vi "WeatherMapAPI_CurrentWeather-Main.vi"() -> (0 "error out":errorcluster, 1 "URL":string, 3 "WeatherMap Current Weather Data":T1)   [LabVIEW 2021]
doc: "Developed By: J Branch\nLast Update: 9/4/2022\n\nDescription: Returns the current weather data to the front panel using the WeatherMap API via HTTP request. The user will need to first navigate to https://openweathermap.org to create an account to get an API key to use the program.\n\nInputs: Zip Code, Country Code\n\nOutput: WeatherMap Current Weather Data Cluster\n\nTo Run: On the block diagram enter the user's API Key into the string text box labelled API Key. Enter the Zip Code and Country Code (us default) in the front panel and select GET Data to execute the API call, the API JSON response will be parsed in the background inside the sub-VIs and formatted to populate the WeatherMap Current Weather Data cluster. \n\nThe Zip Code and County Code can be modified during run-time. \n\nSelect QUIT to terminate the program."
uses:
  <vilib>/httpClient/LabVIEWHTTPClient.lvlib
panel:
  in  "Tab Control":enum32{"User Params", "Internal Params"}(tab)
  out "UserMsg":string
  in  "GetDataButton":bool
  in  "QuitProgramButton":bool
  in  "Zip Code":string
  in  "Country Code":string="us"
  out "HTTP Headers":string
  out "HTTP Body":string
  out "API Key":string="a672f85a4c2930ce00107a5976b7c754"
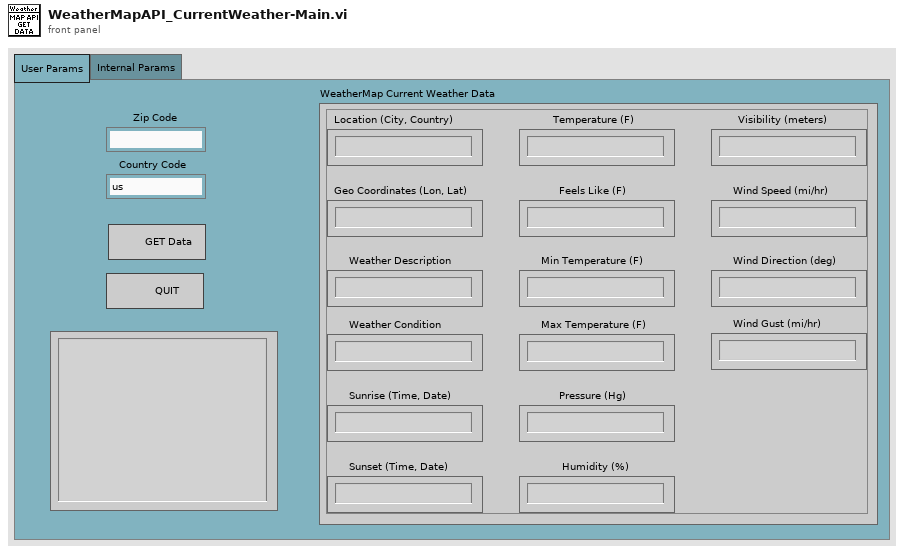
[diagram p1: front panel]
types:
  T1 = cluster{"Location (City, Country)":string, "Geo Coordinates (Lon, Lat)":string, "Weather Description ":string, "Weather Condition":string, "Temperature (F)":string, "Feels Like (F)":string, "Min Temperature (F)":string, "Max Temperature (F)":string, "Pressure (Hg) ":string, "Humidity (%)":string, "Visibility (meters)":string, "Wind Speed (mi/hr)":string, "Wind Direction (deg)":string, "Sunrise (Time, Date)":string, "Sunset (Time, Date)":string, "Wind Gust (mi/hr) ":string}
  T2 = enum8{"Enabled", "Disabled", "Disabled and Grayed Out"}
  T3 = typedef "LabVIEWHTTPClient.lvlib/ClientHandle.ctl" = refnum<k1>
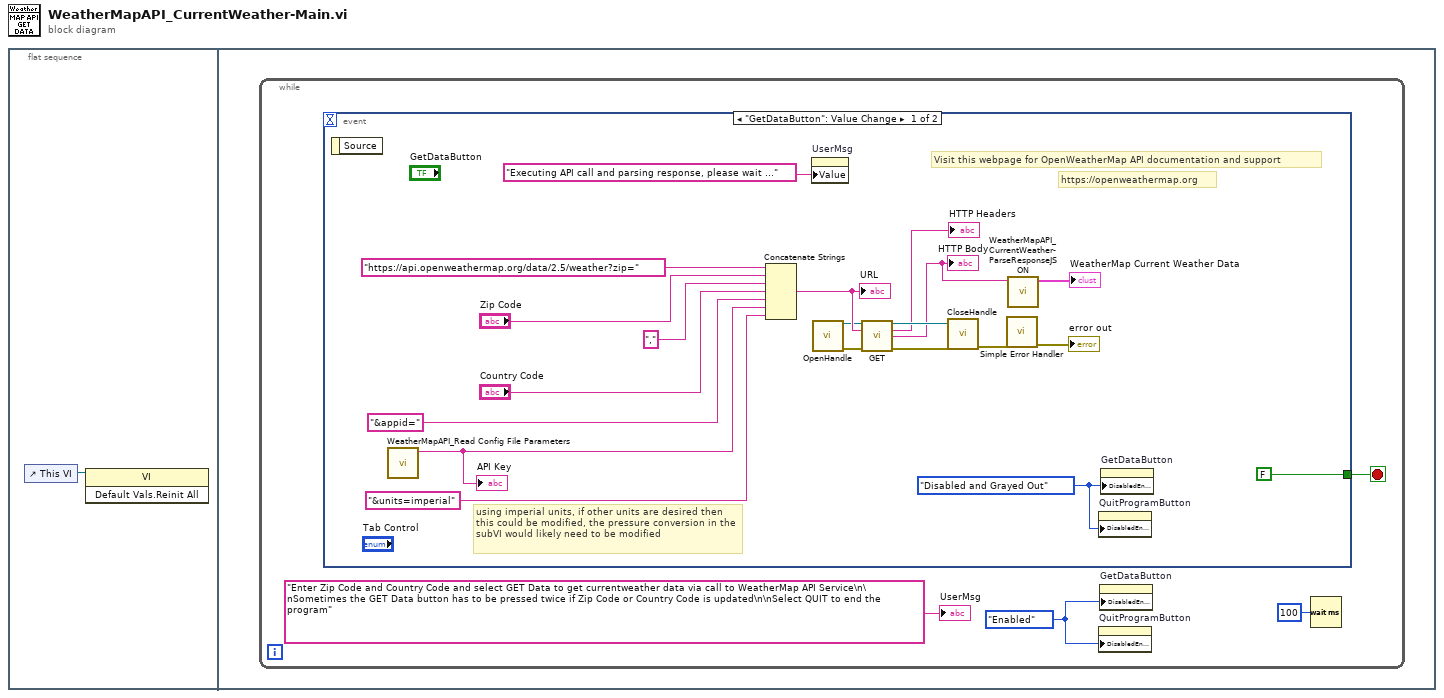
[diagram p0: block diagram]
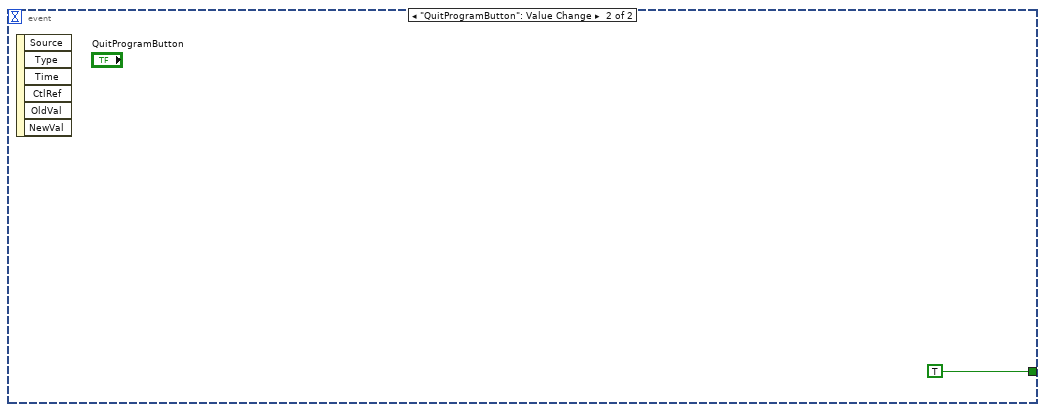
[diagram p2: hidden frame]
diagram:
  n1 = flat-sequence {
    frame #0 {
      n2 = control-ref of="This VI"() -> (w1:refnum<vi>)
      n3 = invoke class="VI" method="Default Vals.Reinit All"(reference=w1) -> ()  [unwired: 2 in, 3 out]
    }
    frame #1 {
      n4 = while {
        stop <- w3 stop-if-true
        w2 = T2."Enabled" ("Disabled")
        n5 = event shown="[0] \"GetDataButton\": Value Change" {
          selector: _ -> [_ _]
          dyn-events: _ -> [_ _]
          timeout: _ -> [_ _]
          tunnel: [FALSE TRUE] -> w3
          event "GetDataButton": Value Change {
            w15 = T2."Disabled and Grayed Out" ("Disabled")
            # "using imperial units, if other units are desired then this could be modified, the pressure conversion in the subVI would likely need to be modified"
            # "Visit this webpage for OpenWeatherMap API documentation and support"
            # "https://openweathermap.org"
            n6 = event-data() -> ()  [unwired: 1 in, 1 out]
            n7 = call "WeatherMapAPI_Read Config File Parameters.vi"() -> ("API Key out"=w6:string)  [unwired: 10 in, 1 out]
            "API Key" <- w6
            n8 = Concatenate Strings("https://api.openweathermap.org/data/2.5/weather?zip=", "Zip Code", ",", "Country Code", "&appid=" ("API Key"), w6, "&units=imperial" ("API Key")) -> (w20:string)
            "URL" <- w20
            n9 = property on="UserMsg" class="Str"("Value"="Executing API call and parsing response, please wait ...") -> ()  [unwired: 2 in, 2 out]
            n10 = call <vilib>:"OpenHandle.vi"() -> ("client handle out"=w14:T3, "error out"=w13:errorcluster)  [unwired: 14 in]
            n11 = call <vilib>:"GET.vi"("client handle"=w14, "url"=w20, "error in (no error)"=w13) -> ("client handle out"=w12:T3, "headers"=→"HTTP Headers":string, "body"=w8:string, "error out"=w11:errorcluster)  [unwired: 9 in]
            "HTTP Body" <- w8
            n12 = call <vilib>:"CloseHandle.vi"("client handle"=w12, "error in (no error)"=w11) -> ("error out"=w9:errorcluster)  [unwired: 13 in]
            n13 = call <vilib>:"Simple Error Handler.vi"("error in (no error)"=w9) -> ("error out"=→"error out":errorcluster)  [unwired: 4 in, 4 out]
            n14 = call "WeatherMapAPI_CurrentWeather-ParseResponseJSON.vi"("API JSON Response"=w8) -> ("WeatherMap Current Weather Data"=→"WeatherMap Current Weather Data":T1)  [unwired: 10 in]
            n15 = property on="QuitProgramButton" class="Bool"("DisabledEnum"=w15) -> ()  [unwired: 2 in, 2 out]
            n16 = property on="GetDataButton" class="Bool"("DisabledEnum"=w15) -> ()  [unwired: 2 in, 2 out]
          }
          event "QuitProgramButton": Value Change {
            n17 = event-data() -> ()  [unwired: 1 in, 6 out]
          }
        }
        n18 = property on="QuitProgramButton" class="Bool"("DisabledEnum"=w2) -> ()  [unwired: 2 in, 2 out]
        n19 = property on="GetDataButton" class="Bool"("DisabledEnum"=w2) -> ()  [unwired: 2 in, 2 out]
        n20 = Wait (ms)(milliseconds to wait=u32 100 ("millisecond multiple")) -> ()  [unwired: 1 out]
        "UserMsg" <- "Enter Zip Code and Country Code and select GET Data to get currentweather data via call to WeatherMap API Service\n\nSometimes the GET Data button has to be pressed twice if Zip Code or Country Code is updated\n\nSelect QUIT to end the program" ("String")
      }
    }
  }
